vi "CallbackTest.vi"() -> ()   [LabVIEW 2025]
uses:
  C:/Users/chrismadlax/Desktop/LVSampleCode/dotNETCallback/netstandard2.0/myClass2.dll
  netstandard2.0/myClass2.dll
panel:
  out "element":string
  in  "SimulateInput":bool
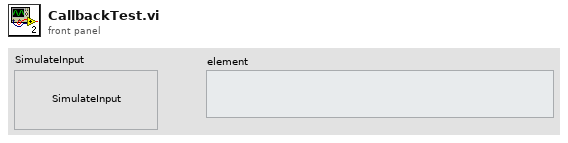
[diagram p1: front panel]
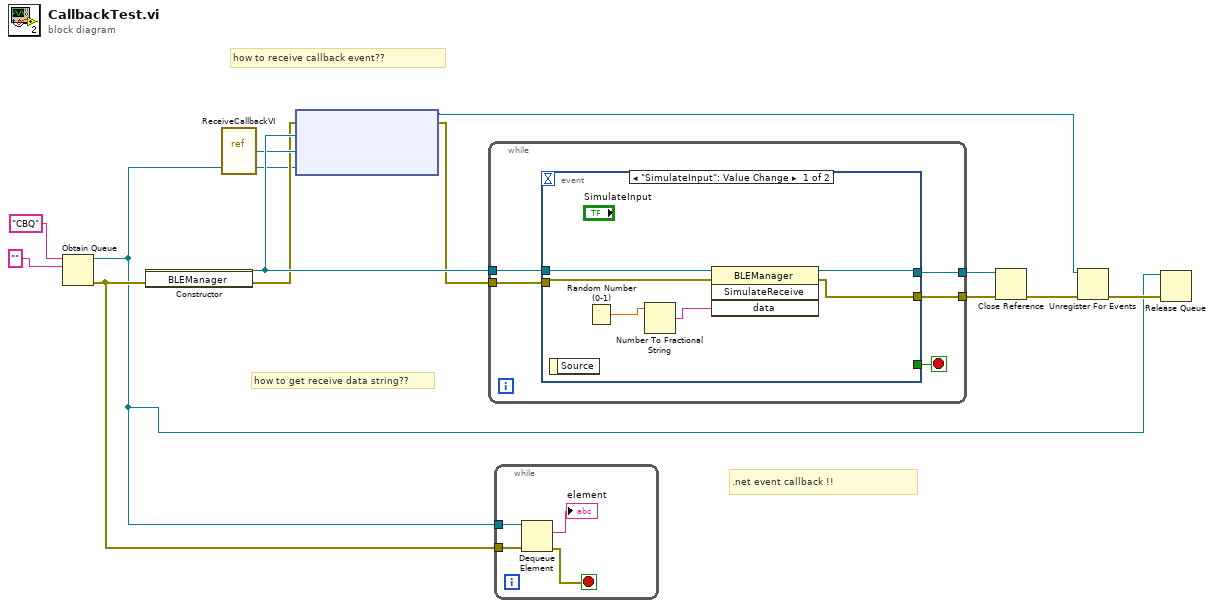
[diagram p0: block diagram]
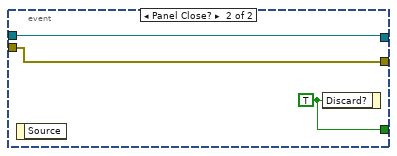
[diagram p2: hidden frame]
diagram:
  # ".net event callback !!"
  # "how to get receive data string??"
  # "how to receive callback event??"
  n1 = Obtain Queue(name (unnamed)="CBQ", element data type="") -> (queue out=w1:refnum<queue>, error out=w2:errorcluster)  [unwired: 3 in, 1 out]
  n2 = constructor class="BLEManager"(error in=w2) -> (reference out=w8:refnum<k24>, error out=w6:errorcluster)  [unwired: 2 in, 1 out]
  n3 = vi-ref "ReceiveCallbackVI.vi"() -> ("vi reference"=w7:refnum<vi>)
  n4 = node(w6, w8, w7, w1) -> (w3:refnum<k27>, w5:errorcluster)  [unwired: 1 in]
  n5 = while {
    tunnel: w5 -> [w18]
    tunnel: w8 -> [w17]
    tunnel: [w16] -> w12
    tunnel: [w15] -> w11
    stop <- w14 stop-if-true
    n6 = event shown="[0] \"SimulateInput\": Value Change" {
      selector: _ -> [_ _]
      dyn-events: _ -> [_ _]
      timeout: _ -> [_ _]
      tunnel: w18 -> [w23 w26]
      tunnel: w17 -> [w24 w27]
      tunnel: [w20 w27] -> w16
      tunnel: [w19 w26] -> w15
      tunnel: [_ w25] -> w14
      event "SimulateInput": Value Change {
        n7 = event-data() -> ()  [unwired: 1 in, 1 out]
        n8 = Random Number (0-1)() -> (number: 0 to 1=w22:dbl)
        n9 = Number To Fractional String(number=w22) -> (F-format string=w21:string)  [unwired: 3 in]
        n10 = invoke class="BLEManager" method="SimulateReceive"(reference=w24, error in=w23, "data"=w21) -> (reference out=w20:refnum<k24>, error out=w19:errorcluster)  [unwired: 1 in, 2 out]
      }
      event Panel Close? {
        w25 = TRUE ("Discard?")
        n11 = event-data() -> ()  [unwired: 1 in, 1 out]
        n12 = event-data("Discard?"=w25) -> ()  [unwired: 1 in, 1 out]
      }
    }
  }
  n13 = while {
    tunnel: w2 -> [w31]
    tunnel: w1 -> [w30]
    stop <- w28 stop-if-true
    n14 = Dequeue Element(queue=w30, error in (no error)=w31) -> (element=→"element":string, error out=w28:errorcluster)  [unwired: 1 in, 2 out]
  }
  n15 = Close Reference(reference=w12, error in (no error)=w11) -> (error out=w10:errorcluster)
  n16 = Unregister For Events(event registration refnum=w3, error in=w10) -> (error out=w4:errorcluster)
  n17 = Release Queue(queue=w1, error in (no error)=w4) -> ()  [unwired: 1 in, 3 out]
